vi "Draw Simple Scale.vi"(7 "heading (rad)":dbl, 9 "Draw Options":T1={"Outer Border Color"=0, "Inner Border Color"=6316128, "Outer Gradient Color"=2565927, "Inner Gradient Color"=16860, "Compass North Pointer Color"=16711680, "Compass Pointer Color 1"=13355429, "Compass Pointer Color 2"=14934973, "Direction Pointer Color"=16765184, "Text Box Outline Color"=13355429, "Text Box Background Color"=14934973, "Scale Color"=16448250, "Text Color"=0, "Draw Gradient"=TRUE, "Draw Rose"=TRUE, "Simple Scale"=TRUE, "Draw Text"=FALSE, "Font Name"="Helvetica", "Angle Units"=enum."Degrees"}, 10 "draw area cache":T3, 11 "picture in":picture) -> (3 "picture out":picture)   [LabVIEW 2017, in "NI_Robotics_Compass Picture.lvlib"]
uses:
  <vilib>/robotics/Controls/Compass Indicator/Compass Picture/NI_Robotics_Compass Picture.lvlib
  <vilib>/robotics/Controls/Compass Indicator/Compass Picture/Draw Area State.ctl
  <vilib>/Utility/miscctls.llb/LVBoundsTypeDef.ctl
  <vilib>/robotics/Controls/Compass Indicator/Compass Picture/Draw Options.ctl
  <vilib>/robotics/Controls/Utilities/Angle Units.ctl
  <vilib>/picture/picture.llb/Draw Text at Point.vi
  <vilib>/picture/picture.llb/Draw Multiple Lines.vi
  <vilib>/Utility/AngleManip/Degrees to Radians (Scalar DBL).vi
  <vilib>/Utility/AngleManip/NI_AngleManipulation.lvlib
  <vilib>/robotics/Controls/Utilities/NI_Robotics_Control Utilities.lvlib
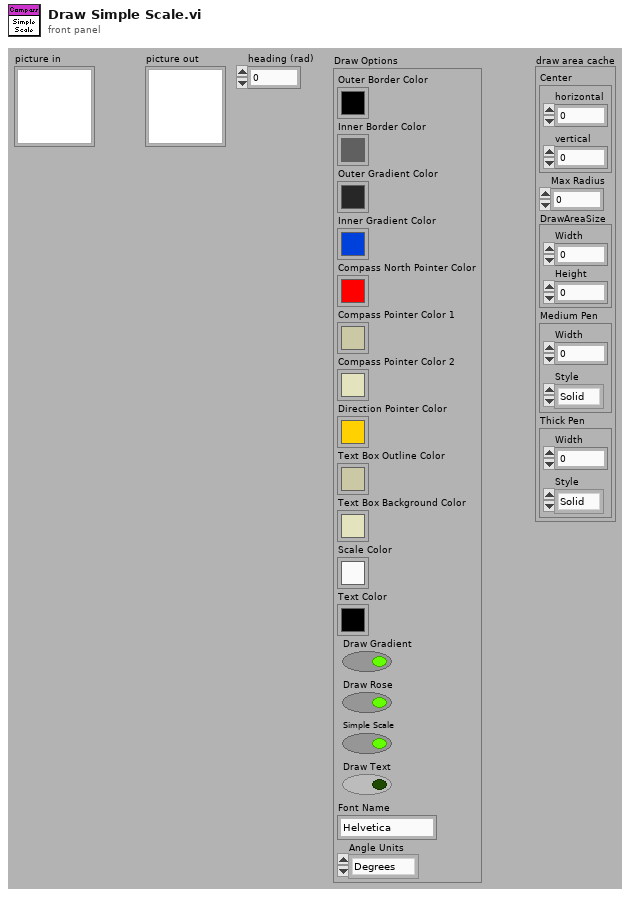
[diagram p1: front panel]
types:
  T1 = typedef "NI_Robotics_Compass Picture.lvlib/Draw Options.ctl" = cluster{"Outer Border Color":u32, "Inner Border Color":u32, "Outer Gradient Color":u32, "Inner Gradient Color":u32, "Compass North Pointer Color":u32, "Compass Pointer Color 1":u32, "Compass Pointer Color 2":u32, "Direction Pointer Color":u32, "Text Box Outline Color":u32, "Text Box Background Color":u32, "Scale Color":u32, "Text Color":u32, "Draw Gradient":bool, "Draw Rose":bool, "Simple Scale":bool, "Draw Text":bool, "Font Name":string, "Angle Units":T2}
  T2 = typedef "NI_Robotics_Control Utilities.lvlib/Angle Units.ctl" = enum16{"Radians", "Degrees"}
  T3 = typedef "NI_Robotics_Compass Picture.lvlib/Draw Area State.ctl" = cluster{"Center":cluster{"horizontal":i16, "vertical":i16}, "Max Radius":dbl, "DrawAreaSize":T4, "Medium Pen":cluster{"Width":u16, "Style":enum32{"Solid", "Dash", "Dot", "DashDot", "DashDotDot"}}, "Thick Pen":cluster{"Width":u16, "Style":enum32{"Solid", "Dash", "Dot", "DashDot", "DashDotDot"}}}
  T4 = typedef "LVBoundsTypeDef.ctl" = cluster{"Width":u32, "Height":u32}
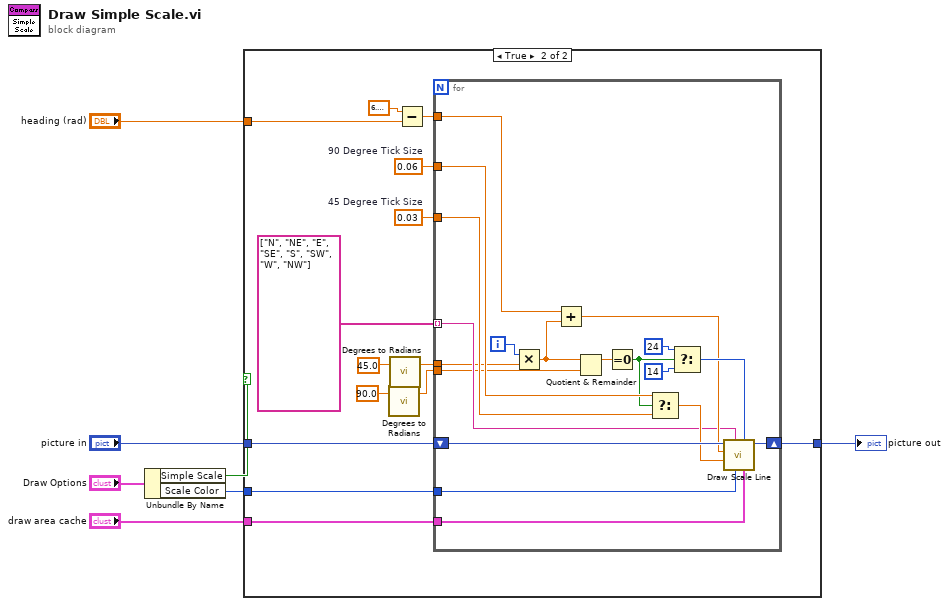
[diagram p0: block diagram]
diagram:
  n1 = Unbundle By Name("Draw Options") -> ("Simple Scale"=w2:bool, "Scale Color"=w1:u32)
  n2 = case shown="True" w2 {
    tunnel: w1 -> [_ w22]
    tunnel: "heading (rad)" -> [_ w20]
    tunnel: "picture in" -> [w8 w17]
    tunnel: [w8 w16] -> w5
    tunnel: "draw area cache" -> [_ w13]
    frame False {
    }
    frame True {
      w15 = 0.06  # 90 Degree Tick Size
      w14 = 0.03  # 45 Degree Tick Size
      n3 = call-poly <vilib>:"Degrees to Radians.vi"("angle (deg)"=90.0 ("y")) -> ("angle (rad)"=w9:dbl)  [unwired: 2 in]
      n4 = call-poly <vilib>:"Degrees to Radians.vi"("angle (deg)"=45.0 ("y")) -> ("angle (rad)"=w11:dbl)  [unwired: 2 in]
      n5 = Subtract(x=6.283185307179586, y=w20) -> (x-y=w21:dbl)
      n6 = for {
        tunnel: w14 -> [w27]
        tunnel: w15 -> [w41]
        shift-right: [w40] -> w16
        shift-left: w17 -> [w39]
        tunnel: string[] ["N", "NE", "E", "SE", "S", "SW", "W", "NW"] -> [w28] mode=indexing
        tunnel: w21 -> [w30]
        tunnel: w22 -> [w29]
        tunnel: w13 -> [w25]
        tunnel: w11 -> [w24]
        tunnel: w9 -> [w23]
        i -> [w37]
        n7 = Multiply(x=w37, y=w24) -> (x*y=w32:dbl)
        n8 = Add(x=w30, y=w32) -> (x+y=w31:dbl)
        n9 = Quotient & Remainder(x=w32, y=w23) -> (x-y*floor(x/y)=w36:dbl)  [unwired: 1 out]
        n10 = Equal To 0?(x=w36) -> (x = 0?=w26:bool)
        n11 = Select(t=w41, s=w26, f=w27) -> (s? t:f=w38:dbl)
        n12 = Select(t=24 ("y"), s=w26, f=14 ("y")) -> (s? t:f=w35:i32)
        n13 = call <vilib>:"Draw Scale Line.vi"("draw area cache"=w25, "font size"=w35, "scale color"=w29, "scale label"=w28, "line size (0-1)"=w38, "heading (rad)"=w31, "picture in"=w39) -> ("picture out"=w40:picture)  [unwired: 4 in]
      }
    }
  }
  "picture out" <- w5
